vi "7.3.Telegram_Relay_Control_Read Temp.vi"   [LabVIEW 2014]
uses:
  <vilib>/Aledyne-TSXperts/Arduino Compatible Compiler for LabVIEW/Code Generator/Arduino APIs/Digital/PinDirection.ctl
  <vilib>/Aledyne-TSXperts/Arduino Compatible Compiler for LabVIEW/addons/QwaveSys_ESP8266/QwaveSys_ESP8266.lvlib
  <vilib>/Aledyne-TSXperts/Arduino Compatible Compiler for LabVIEW/Arduino Compatible Compiler for LabVIEW.lvlib
  <vilib>/Aledyne-TSXperts/Arduino Compatible Compiler for LabVIEW/addons/QwaveSys_Interface/QwaveSys_Interface.lvlib
types:
  T1 = typedef "Arduino Compatible Compiler for LabVIEW.lvlib/PinDirection.ctl" = enum16{" INPUT", "OUTPUT", " INPUT_PULLUP"}
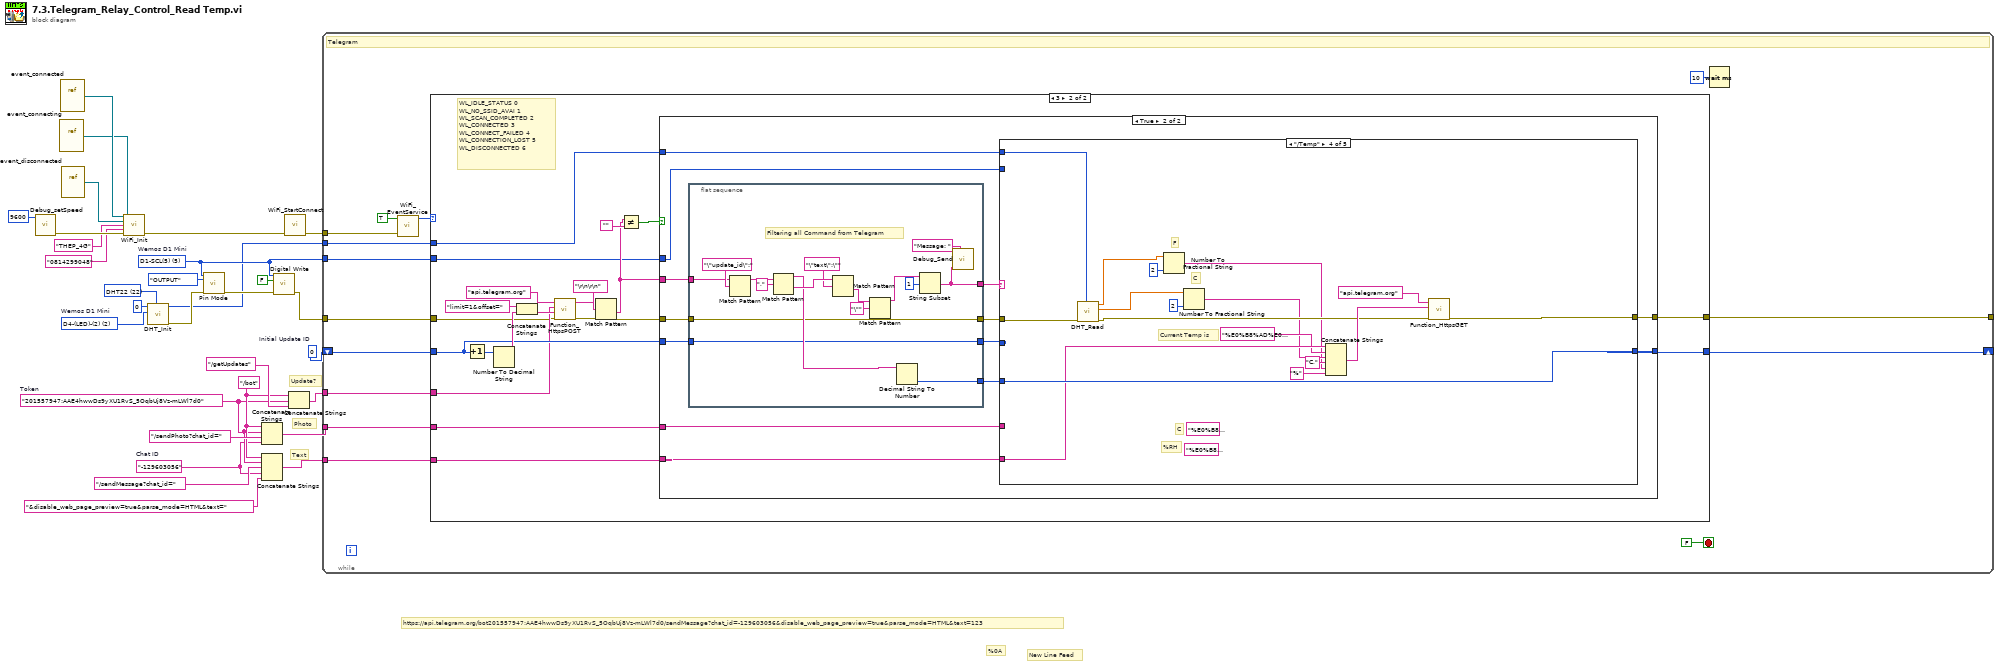
[diagram p0: block diagram]
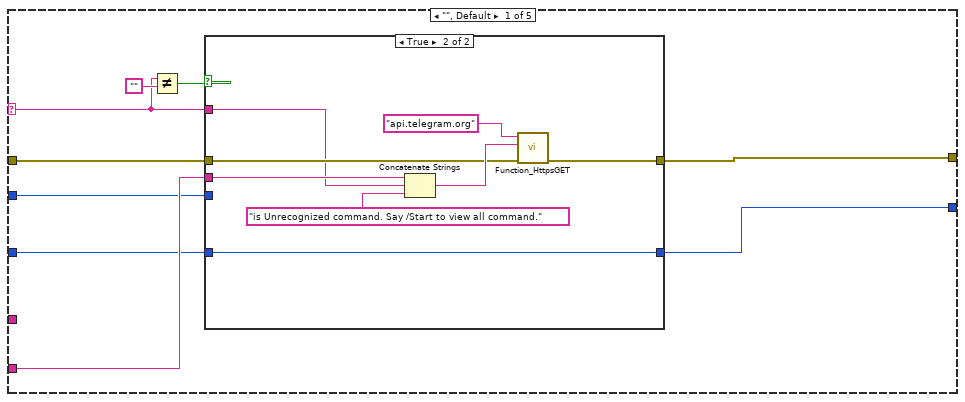
[diagram p4: hidden frame]
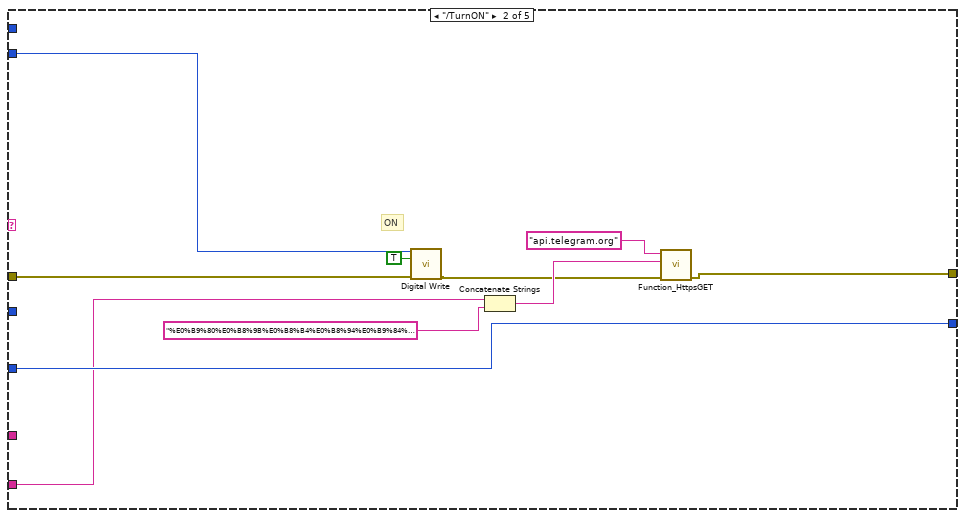
[diagram p6: hidden frame]
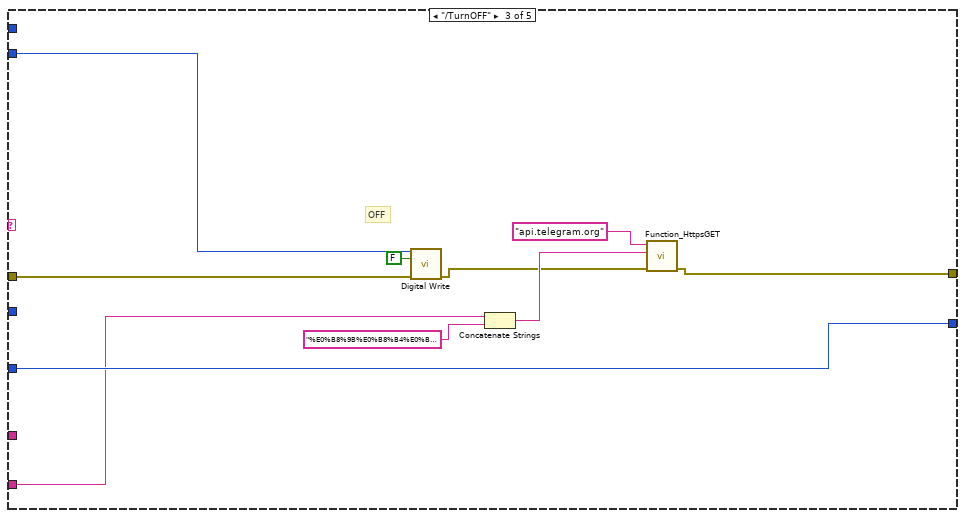
[diagram p7: hidden frame]
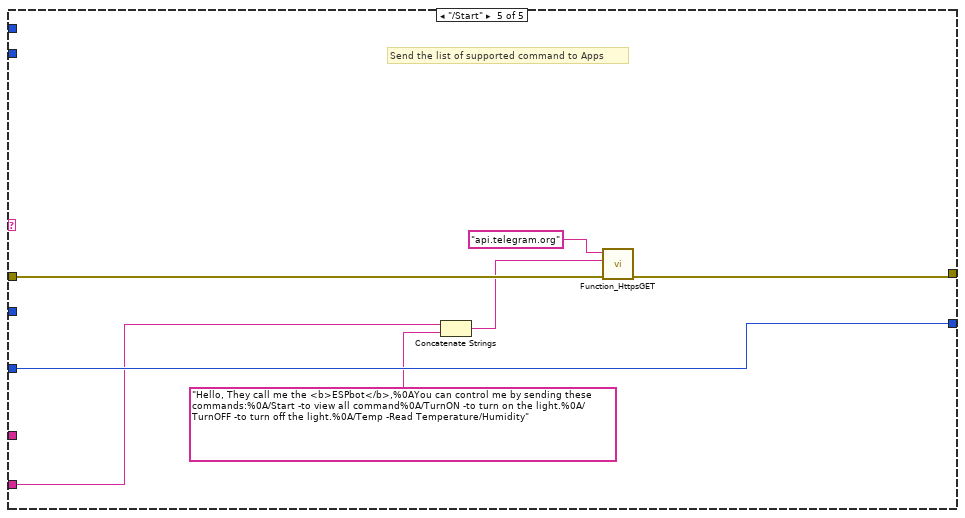
[diagram p8: hidden frame]
diagram:
  w1 = u8 2 items=["D0-(16)"=16, "D1-SCL(5)"=5, "D2-SDA(4)"=4, "D3-(0)"=0, "D4-(LED)-(2)"=2, "D5-SCK(14)"=14, "D6-MISO(12)"=12, "D7-MOSI(13)"=13, "D8-SS(15)"=15, "TX(3)"=3, "RX(1)"=1, "ADC0,(17)"=17]  # Wemos D1 Mini
  w3 = u16 22 items=["DHT11"=11, "DHT21"=21, "DHT22"=22] ("Type")
  w7 = u8 5 items=["D0-(16)"=16, "D1-SCL(5)"=5, "D2-SDA(4)"=4, "D3-(0)"=0, "D4-(LED)-(2)"=2, "D5-SCK(14)"=14, "D6-MISO(12)"=12, "D7-MOSI(13)"=13, "D8-SS(15)"=15, "TX(3)"=3, "RX(1)"=1, "ADC0,(17)"=17]  # Wemos D1 Mini
  w19 = 0  # Initial Update ID
  w16 = "201557947:AAE4hwwDs9yXU1RvS_5OqbUj8Vz-mLWl7d0"  # Token
  w17 = "/bot"
  w14 = "-129603056"  # Chat ID
  # "New Line Feed"
  # "%0A"
  # "https://api.telegram.org/bot201557947:AAE4hwwDs9yXU1RvS_5OqbUj8Vz-mLWl7d0/sendMessage?chat_id=-129603056&disable_web_page_preview=true&parse_mode=HTML&text=123"
  # "Update?"
  # "Photo"
  # "Text"
  n1 = call <vilib>:"Debug_setSpeed.vi"("Speed"=u32 9600) -> ("error out"=w29:errorcluster)  [unwired: 10 in]
  n2 = vi-ref "event_connecting.vi"() -> (w25:refnum<vi>)
  n3 = vi-ref "event_connected.vi"() -> (w26:refnum<vi>)
  n4 = vi-ref "event_disconnected.vi"() -> (w24:refnum<vi>)
  n5 = call <vilib>:"WiFi_Init.vi"("connected"=w26, "connecting"=w25, "disconnected"=w24, "SSID"="THEP_4G", "PASSPHARSE"="0814299048", "error in (no error)"=w29) -> ("error out"=w6:errorcluster)  [unwired: 9 in]
  n6 = call <vilib>:"DHT_Init.vi"("Type"=w3, "PIN"=w1, "Interface (0-4)"=u8 0) -> ("error out"=w5:errorcluster, "Instance"=w4:u8)  [unwired: 7 in]
  n7 = call <vilib>:"Pin Mode.vi"("pin"=w7, "direction"=PinDirection."OUTPUT", "error in (no error)"=w5) -> ("error out"=w10:errorcluster)  [unwired: 12 in]
  n8 = Concatenate Strings(w17, w16, "/sendPhoto?chat_id=", w14) -> (w18:string)
  n9 = Concatenate Strings(w17, w16, "/sendMessage?chat_id=", w14, "&disable_web_page_preview=true&parse_mode=HTML&text=") -> (w13:string)
  n10 = call <vilib>:"Digital Write.vi"("pin"=w7, "state"=FALSE, "error in (no error)"=w10) -> ("error out"=w9:errorcluster)  [unwired: 12 in]
  n11 = call <vilib>:"WiFi_StartConnect.vi"("error in (no error)"=w6) -> ("error out"=w30:errorcluster)  [unwired: 10 in]
  n12 = Concatenate Strings(w17, w16, "/getUpdates") -> (w20:string)
  n13 = while {
    tunnel: w30 -> [w43]
    tunnel: w18 -> [w38]
    tunnel: w20 -> [w39]
    shift-right: [w37] -> _
    shift-left: w19 -> [w40]
    tunnel: [w36] -> _
    tunnel: w13 -> [w34]
    tunnel: w9 -> [w33]
    tunnel: w7 -> [w32]
    tunnel: w4 -> [w31]
    stop <- FALSE stop-if-true
    # "Telegram"
    n14 = call <vilib>:"WiFi_EventService.vi"("error in (no error)"=w43, "wait for connected (True)"=TRUE) -> ("Status"=w35:u16)  [unwired: 8 in, 1 out]
    n15 = case shown="3" w35 {
      tunnel: w40 -> [w46 w53]
      tunnel: w39 -> [_ w52]
      tunnel: w38 -> [_ w60]
      tunnel: [w46 w59] -> w37
      tunnel: [w45 w58] -> w36
      tunnel: w34 -> [_ w57]
      tunnel: w33 -> [w45 w49]
      tunnel: w32 -> [_ w48]
      tunnel: w31 -> [_ w47]
      frame 0, Default {
      }
      frame 3 {
        # "WL_IDLE_STATUS\t0\nWL_NO_SSID_AVAI\t1\nWL_SCAN_COMPLETED\t2\nWL_CONNECTED\t3\nWL_CONNECT_FAILED\t4\nWL_CONNECTION_LOST\t5\nWL_DISCONNECTED\t6"
        n16 = Increment(x=w53) -> (x+1=w54:i32)
        n17 = Number To Decimal String(number=w54) -> (decimal integer string=w66:string)  [unwired: 1 in]
        n18 = Concatenate Strings("limit=1&offset=", w66) -> (w64:string)
        n19 = call <vilib>:"Function_HttpsPOST.vi"("error in (no error)"=w49, "DATA"=w64, "URI"=w52, "Host"="api.telegram.org") -> ("error out"=w61:errorcluster, "Results"=w55:string)  [unwired: 6 in]
        n20 = Match Pattern(string=w55, regular expression="\r\n\r\n") -> (after substring=w50:string)  [unwired: 1 in, 3 out]
        n21 = Not Equal?(x=w50, y="") -> (x != y?=w51:bool)
        n22 = case shown="True" w51 {
          tunnel: w50 -> [_ w75]
          tunnel: w61 -> [w68 w79]
          tunnel: [w68 w81] -> w58
          tunnel: w60 -> [_ w80]
          tunnel: [w67 w73] -> w59
          tunnel: w57 -> [_ w76]
          tunnel: w53 -> [w67 w72]
          tunnel: w48 -> [_ w70]
          tunnel: w47 -> [_ w69]
          frame False {
          }
          frame True {
            n23 = flat-sequence {
              tunnel: [w89] -> w74
              tunnel: w79 -> [w88]
              tunnel: [w88] -> w78
              tunnel: [w85] -> w77
              tunnel: w75 -> [w84]
              tunnel: [w82] -> w71
              tunnel: w72 -> [w82]
              frame #0 {
                # "Filtering all Command from Telegram"
                n24 = Match Pattern(string=w84, regular expression="\"update_id\":") -> (after substring=w92:string)  [unwired: 1 in, 3 out]
                n25 = Match Pattern(string=w92, regular expression=",") -> (before substring=w90:string, after substring=w97:string)  [unwired: 1 in, 2 out]
                n26 = Match Pattern(string=w97, regular expression="\"text\":\"") -> (after substring=w95:string)  [unwired: 1 in, 3 out]
                n27 = Match Pattern(string=w95, regular expression="\"") -> (before substring=w86:string)  [unwired: 1 in, 3 out]
                n28 = Decimal String To Number(string=w90) -> (number=w89:i32)  [unwired: 2 in, 1 out]
                n29 = String Subset(string=w86, offset (0)=1) -> (substring=w85:string)  [unwired: 1 in]
                n30 = call <vilib>:"Debug_Send.vi"("Name"="Message: ", "DATA"=w85) -> ()  [unwired: 10 in]
              }
            }
            n31 = case shown="\"/Temp\"" w77 {
              selector: w77 -> [w98 _ _ _ _]
              tunnel: w78 -> [w106 w126 w136 w148 w159]
              tunnel: w80 -> [_ _ _ _ _]
              tunnel: [w105 w117 w128 w149 w158] -> w81
              tunnel: w76 -> [w104 w119 w130 w150 w155]
              tunnel: w74 -> [w101 w123 w133 w153 w157]
              tunnel: [w100 w123 w133 w153 w157] -> w73
              tunnel: w71 -> [w99 _ _ _ _]
              tunnel: w70 -> [_ w125 w135 _ _]
              tunnel: w69 -> [_ _ _ w147 _]
              frame "", Default {
                n32 = Not Equal?(x=w98, y="" ("Empty String Constant")) -> (x != y?=w102:bool)
                n33 = case shown="True" w102 {
                  tunnel: w106 -> [w108 w114]
                  tunnel: [w108 w113] -> w105
                  tunnel: w104 -> [_ w112]
                  tunnel: w98 -> [_ w111]
                  tunnel: w101 -> [_ w109]
                  tunnel: [w107 w109] -> w100
                  tunnel: w99 -> [w107 _]
                  frame False {
                  }
                  frame True {
                    n34 = Concatenate Strings(w112, w111, "is Unrecognized command. Say /Start to view all command." ("string")) -> (w115:string)
                    n35 = call <vilib>:"Function_HttpsGET.vi"("error in (no error)"=w114, "URI"=w115, "Host"="api.telegram.org") -> ("error out"=w113:errorcluster)  [unwired: 7 in, 1 out]
                  }
                }
              }
              frame "/TurnON" {
                # "ON"
                n36 = call <vilib>:"Digital Write.vi"("pin"=w125, "state"=TRUE, "error in (no error)"=w126) -> ("error out"=w120:errorcluster)  [unwired: 12 in]
                n37 = Concatenate Strings(w119, "%E0%B9%80%E0%B8%9B%E0%B8%B4%E0%B8%94%E0%B9%84%E0%B8%9F%E0%B9%83%E0%B8%AB%E0%B9%89%E0%B9%81%E0%B8%A5%E0%B9%89%E0%B8%A7%E0%B8%84%E0%B9%88%E0%B8%B0...") -> (w121:string)
                n38 = call <vilib>:"Function_HttpsGET.vi"("error in (no error)"=w120, "URI"=w121, "Host"="api.telegram.org") -> ("error out"=w117:errorcluster)  [unwired: 7 in, 1 out]
              }
              frame "/TurnOFF" {
                # "OFF"
                n39 = call <vilib>:"Digital Write.vi"("pin"=w135, "state"=FALSE, "error in (no error)"=w136) -> ("error out"=w129:errorcluster)  [unwired: 12 in]
                n40 = Concatenate Strings(w130, "%E0%B8%9B%E0%B8%B4%E0%B8%94%E0%B9%84%E0%B8%9F%E0%B9%81%E0%B8%A5%E0%B9%89%E0%B8%A7%E0%B8%84%E0%B9%88%E0%B8%B0%21") -> (w131:string)
                n41 = call <vilib>:"Function_HttpsGET.vi"("error in (no error)"=w129, "URI"=w131, "Host"="api.telegram.org") -> ("error out"=w128:errorcluster)  [unwired: 7 in, 1 out]
              }
              frame "/Temp" {
                (unwired) "%E0%B8%84%E0%B8%A7%E0%B8%B2%E0%B8%A1%E0%B8%8A%E0%B8%B7%E0%B9%89%E0%B8%99%E0%B8%AA%E0%B8%B1%E0%B8%A1%E0%B8%9E%E0%B8%B1%E0%B8%97%E0%B8%98%E0%B9%8C"
                (unwired) "%E0%B8%AD%E0%B8%87%E0%B8%A8%E0%B8%B2%E0%B9%80%E0%B8%8B%E0%B8%A5%E0%B9%80%E0%B8%8B%E0%B8%B5%E0%B8%A2%E0%B8%AA"
                # "F"
                # "%RH"
                # "C"
                # "C"
                # "Current Temp is"
                n42 = call <vilib>:"DHT_Read.vi"("Instance"=w147, "error in (no error)"=w148) -> ("error out"=w146:errorcluster, "Celsius"=w145:dbl, "Humidity"=w141:dbl)  [unwired: 4 in, 3 out]
                n43 = Number To Fractional String(number=w141, precision (6)=i16 2) -> (F-format string=w139:string)  [unwired: 2 in]
                n44 = Number To Fractional String(number=w145, precision (6)=i16 2) -> (F-format string=w143:string)  [unwired: 2 in]
                n45 = Concatenate Strings(w150, "%E0%B8%AD%E0%B8%B8%E0%B8%93%E0%B8%AB%E0%B8%A0%E0%B8%B9%E0%B8%A1%E0%B8%B4%E0%B8%82%E0%B8%93%E0%B8%B0%E0%B8%99%E0%B8%B5%E0%B9%89%E0%B8%84%E0%B8%B7%E0%B8%AD+", w143, "C," ("string"), w139, "%" ("string")) -> (w151:string)
                n46 = call <vilib>:"Function_HttpsGET.vi"("error in (no error)"=w146, "URI"=w151, "Host"="api.telegram.org") -> ("error out"=w149:errorcluster)  [unwired: 7 in, 1 out]
              }
              frame "/Start" {
                # "Send the list of supported command to Apps"
                n47 = Concatenate Strings(w155, "Hello, They call me the <b>ESPbot</b>,%0AYou can control me by sending these commands:%0A/Start -to view all command%0A/TurnON -to turn on the light.%0A/TurnOFF -to turn off the light.%0A/Temp -Read Temperature/Humidity") -> (w156:string)
                n48 = call <vilib>:"Function_HttpsGET.vi"("error in (no error)"=w159, "URI"=w156, "Host"="api.telegram.org") -> ("error out"=w158:errorcluster)  [unwired: 7 in, 1 out]
              }
            }
          }
        }
      }
    }
    n49 = Wait (ms)(milliseconds to wait=u32 10) -> ()  [unwired: 1 out]
  }
